vi "Demo- Rename document from list.vi"() -> ()   [LabVIEW 2019]
panel:
  out "element":string
  out "Numeric":i32
  out "Ring 2":u16(ring) items=["somethingotherthantest", "milandd", "test", "milan", "latest doc", "renamed name", "milan", "latest doc", "milan", "latest doc", "milan", "qq1", "qq", "HELLO MILAN boss", "very cool", "HELLO MILAN", "new", "OnShape_Placemat_Glasses Challenge.pdf", "Untitled document", "FeatureStudio Test"]
  in  "OK Button":bool
  in  "Ring":u16(ring) items=["somethingotherthantest", "milandd", "test", "milan", "latest doc", "renamed name", "milan", "latest doc", "milan", "latest doc", "milan", "qq1", "qq", "HELLO MILAN boss", "very cool", "HELLO MILAN", "new", "OnShape_Placemat_Glasses Challenge.pdf", "Untitled document", "FeatureStudio Test"]
  out "List of Documents":string[][](array[string])
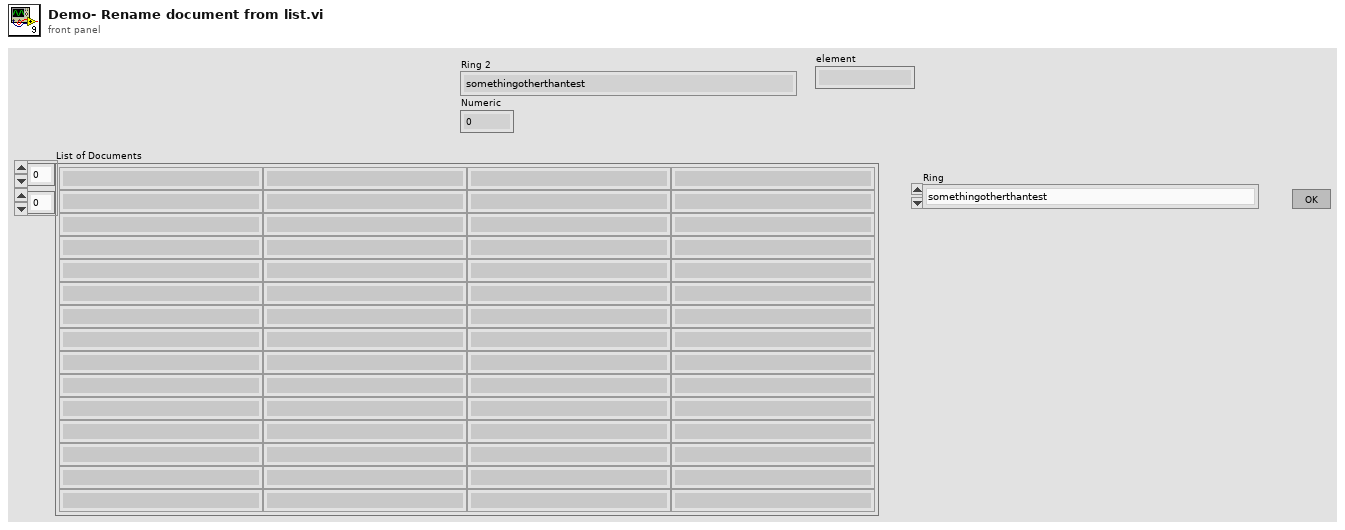
[diagram p1: front panel]
types:
  T1 = typedef "Cluster.ctl" = cluster{"Date":string, "On-Nonce":string, "eid":string, "wid":string, "did":string, "name":string, "method":string, "Accept":string, "User-Agent":string, "Content-Type":string, "stack":string, "headers":string[], "payload":string, "ctype":string, "path":string, "Authorization":string, "secret_key":string, "access_key":string}
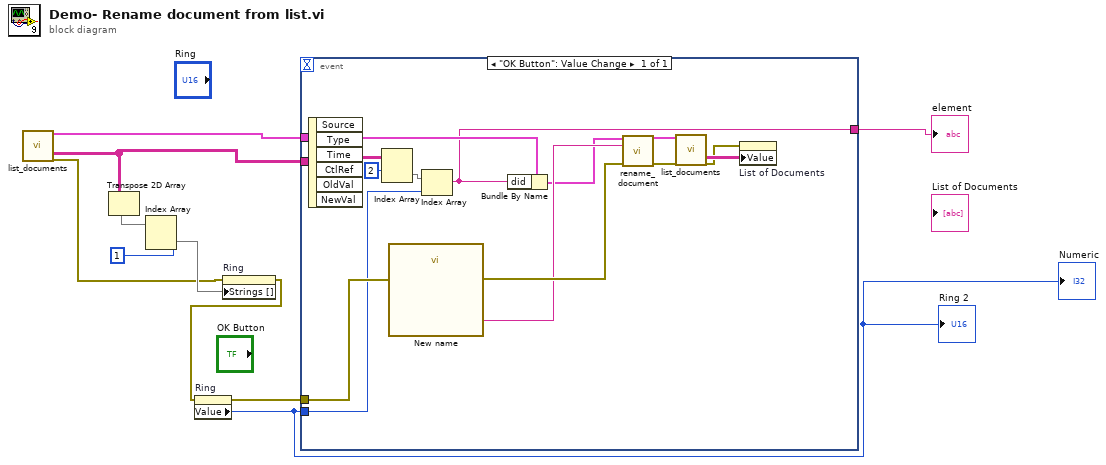
[diagram p0: block diagram]
diagram:
  n1 = call "list_documents.vi"() -> ("Device Out"=w10:T1, "Document list"=w9:string[][], "error out"=w5:errorcluster)  [unwired: 16 in, 1 out]
  n2 = Transpose 2D Array(2D array=w9) -> (transposed array=w8:string[][])
  n3 = Index Array(array=w8, index (row)=1) -> (element=w6:string[])  [unwired: 1 in]
  n4 = property on="Ring" class="Ring (strict)"(error in=w5, "Strings []"=w6) -> (error out=w4:errorcluster)  [unwired: 1 in, 1 out]
  n5 = property on="Ring" class="Ring (strict)"(error in=w4) -> (error out=w3:errorcluster, "Value"=w2:u16)  [unwired: 1 in, 1 out]
  "Ring 2" <- w2
  "Numeric" <- w2
  n6 = event shown="[0] \"OK Button\": Value Change" {
    selector: _ -> [_]
    dyn-events: _ -> [_]
    timeout: _ -> [_]
    tunnel: w10 -> [w21]
    tunnel: w9 -> [w16]
    tunnel: w3 -> [w13]
    tunnel: w2 -> [w12]
    tunnel: [w11] -> w1
    event "OK Button": Value Change {
      n7 = event-data() -> ()  [unwired: 1 in, 6 out]
      n8 = Index Array(array=w16, index (row)=2) -> (element=w17:string[])  [unwired: 1 in]
      n9 = call "New name"("error in (no error)"=w13) -> ("New name"=w22:string, "error out"=w23:errorcluster)  [unwired: 16 in, 1 out]
      n10 = Index Array(array=w17, index=w12) -> (element=w11:string)
      n11 = Bundle By Name(cluster=w21, "did"=w11) -> (w20:T1)
      n12 = call "rename_document.vi"("Device In"=w20, "New Name"=w22, "error in"=w23) -> ("Device Out"=w19:T1, "error out"=w24:errorcluster)  [unwired: 10 in, 1 out]
      n13 = call "list_documents.vi"("Device In"=w19, "error in"=w24) -> ("Document list"=w18:string[][], "error out"=w15:errorcluster)  [unwired: 14 in, 2 out]
      n14 = property on="List of Documents" class="Arr (strict)"(error in=w15, "Value"=w18) -> ()  [unwired: 1 in, 2 out]
    }
  }
  "element" <- w1
